vi "linspace.vi"(1 "N":i32=1, 2 "end":dbl=10.0, 3 "start":dbl) -> (0 "X":dbl[](array[numeric]))   [LabVIEW 2021]
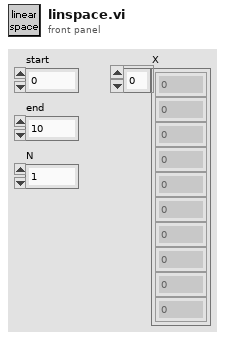
[diagram p1: front panel]
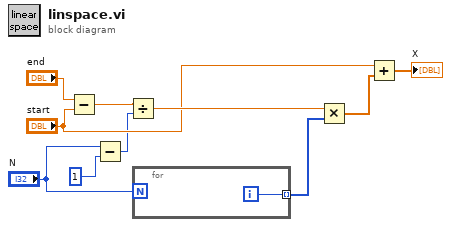
[diagram p0: block diagram]
diagram:
  n1 = Subtract(x="end", y="start") -> (x-y=w9:dbl)
  n2 = Subtract(x="N", y=1) -> (x-y=w2:i32)
  n3 = Divide(x=w9, y=w2) -> (x/y=w7:dbl)
  n4 = for {
    N: "N" -> [_]
    tunnel: [w11] -> w8 mode=indexing
    i -> [w11]
  }
  n5 = Multiply(x=w7, y=w8) -> (x*y=w5:dbl[])
  n6 = Add(x="start", y=w5) -> (x+y=→"X":dbl[])
